vi "NI VeriStand - Set Custom Device Driver.vi"(7 "Execution mode":T3, 8 "error in (no error)":errorcluster, 9 "Driver VI Path (Host)":T1, 10 "Driver VI Path (RT)":path, 11 "Device Ref in":T4 format="%.0x") -> (0 "error out":errorcluster, 3 "Device Ref out":T4 format="%.0x")   [LabVIEW 2020, in "Custom Device API.lvlib"]
doc: "LabVIEW no longer supports this VI. Use the NI VeriStand - Set Custom Device Drivers VI instead.\n\nSpecifies the execution mode and paths of the custom device driver VI. Use this VI to programmatically change the driver library for a custom device, which can be necessary if the device runs on multiple operating systems that require different driver VIs, or if the device runs in different execution modes (for example, Inline HW Interface and Asynchronous).\n\n<B>Note:</B> You must base the driver VI on the template associated with the specified <B>Execution mode</B>. You can configure the driver VI only when you configure the device. The user cannot update the driver VI at run time."
uses:
  <vilib>/NI VeriStand/Custom Device API/Custom Device API.lvlib
  <vilib>/NI VeriStand/Custom Device API/Custom Device Item Ref.ctl
  <vilib>/NI VeriStand/Custom Device API/Custom Device Execution Mode.ctl
  <vilib>/NI VeriStand/Custom Device API/Path Specification.ctl
  <vilib>/NI VeriStand/Custom Device API/Path Type.ctl
  <vilib>/NI VeriStand/Custom Device API/Custom Device Supported Target.ctl
  <vilib>/NI VeriStand/Custom Device API/Custom Device Path Data.ctl
  e9e63dab-a62c-46fe-a4e7-fed09df0bc62.vi
  <vilib>/NI VeriStand/Custom Device API/Custom Device Offline Path.vi
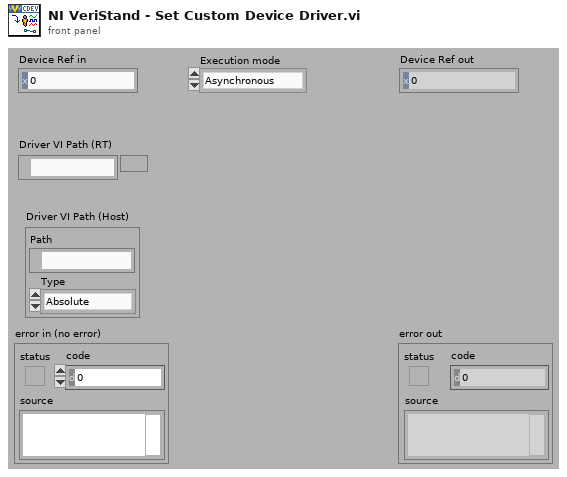
[diagram p1: front panel]
types:
  T1 = typedef "Custom Device API.lvlib/Path Specification.ctl" = cluster{"Path":path, "Type":T2}
  T2 = typedef "Custom Device API.lvlib/Path Type.ctl" = enum16{"Absolute", "To Base", "To Common Data Dir", "To Application Data Dir"}
  T3 = typedef "Custom Device API.lvlib/Custom Device Execution Mode.ctl" = enum16{"Asynchronous", "Inline HW Interface", "Inline Model Interface", "Inline Timing and Sync", "Asynchronous Timing and Sync"}
  T4 = typedef "Custom Device API.lvlib/Custom Device Item Ref.ctl" = u64
  T5 = typedef "Custom Device API.lvlib/Custom Device Supported Target.ctl" = enum16{"All", "PharLap", "VxWorks", "Windows", "Linux_32_ARM", "Linux_x64", "PharLap & Windows", "PharLap & VxWorks", "VxWorks & Windows"}
  T6 = typedef "Custom Device API.lvlib/Custom Device Path Data.ctl" = cluster{"SupportedTarget":T5, "Source":T1, "RT Destination":path}
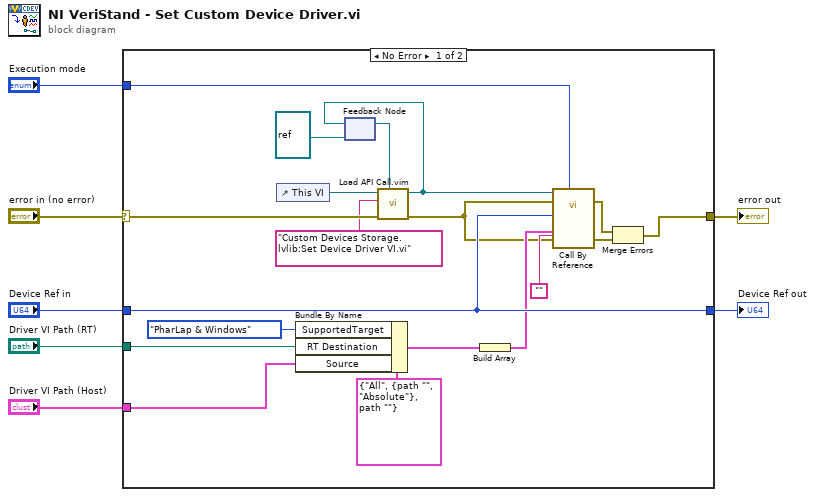
[diagram p0: block diagram]
diagram:
  n1 = case shown="No Error" "error in (no error)" {
    selector: "error in (no error)" -> [w13 w28]
    tunnel: "Execution mode" -> [w25 _]
    tunnel: "Device Ref in" -> [w17 w27]
    tunnel: [w24 w28] -> w5
    tunnel: [w17 w27] -> w4
    tunnel: "Driver VI Path (Host)" -> [w20 _]
    tunnel: "Driver VI Path (RT)" -> [w19 _]
    frame No Error {
      n2 = control-ref of="This VI"() -> (w14:refnum<vi>)
      n3 = Bundle By Name(cluster=T6 {"SupportedTarget"=enum."All", "Source"={"Path"=path "", "Type"=enum."Absolute"}, "RT Destination"=path ""} ("Driver VI Path"), "SupportedTarget"=Custom_Device_Supported_Target."PharLap & Windows", "RT Destination"=w19, "Source"=w20) -> (w18:T6)
      n4 = feedback #1(refnum<vi> refnum ("type specifier VI Refnum (for type only)")) -> (w15:refnum<vi>)
      n5 = call "Load API Call.vim"("VI reference in"=w15, "error in (no error)"=w13, "VI qualified name"="Custom Devices Storage.lvlib:Set Device Driver VI.vi", "Caller VI ref"=w14) -> ("error out"=w12:errorcluster, "VI reference"=w11:refnum<vi>)  [unwired: 6 in]
      n6 = feedback-in #1(w11) -> ()
      n7 = Build Array(w18) -> (w16:T6[])
      n8 = call-by-ref "?"(reference=w11, error in=w12, "Version"="", "Execution mode"=w25, 8:"error in (no error)"=w12, "Driver VI"=w16, "Device Ref in"=w17) -> (error out=w8:errorcluster, 0:"error out"=w26:errorcluster)  [unwired: 5 in, 2 out]
      n9 = Merge Errors(w8, w26) -> (w24:errorcluster)
    }
    frame Error {
    }
  }
  "Device Ref out" <- w4
  "error out" <- w5
